vi "Mod N Indexer  U16.vi"(6 "reset":bool=TRUE, 8 "enable":bool=TRUE, 9 "reset value":u16, 10 "N":u16, 11 "initial value":u16) -> (0 "index zero":bool, 1 "next index":u16, 2 "index":u16, 3 "wrap back":bool)   [LabVIEW 2020]
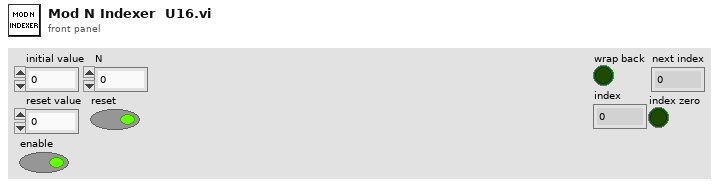
[diagram p1: front panel]
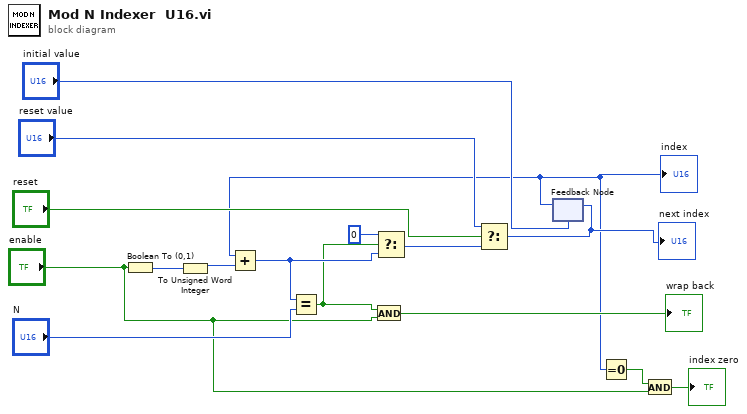
[diagram p0: block diagram]
diagram:
  n1 = Boolean To (0,1)(Boolean="enable") -> (0, 1=w16:i16)
  n2 = To Unsigned Word Integer(number=w16) -> (unsigned 16bit integer=w15:u16)
  n3 = feedback #1("initial value") -> (w1:u16)
  "index" <- w1
  n4 = Add(x=w1, y=w15) -> (x+y=w13:u16)
  n5 = Equal?(x=w13, y="N") -> (x = y?=w11:bool)
  n6 = And(x=w11, y="enable") -> (x .and. y?=→"wrap back":bool)
  n7 = Select(t=u16 0, s=w11, f=w13) -> (s? t:f=w12:u16)
  n8 = Select(t="reset value", s="reset", f=w12) -> (s? t:f=w9:u16)
  "next index" <- w9
  n9 = feedback-in #1(w9) -> ()
  n10 = Equal To 0?(x=w1) -> (x = 0?=w8:bool)
  n11 = And(x=w8, y="enable") -> (x .and. y?=→"index zero":bool)
